vi "Error Handler.vi"(8 "error in":errorcluster, 10 "state":T1=enum."Start", 11 "dispatcher in":refnum<class "Dispatcher Thread.lvclass">) -> (0 "error out":errorcluster, 3 "dispatcher out":refnum<class "Dispatcher Thread.lvclass">)   [LabVIEW 2019, in "DSF Core.lvlib" / "Dispatcher Thread.lvclass"]
uses:
  Dispatcher Thread.lvclass
  Interface/Dispatcher/Command.ctl
  Interface/Dispatcher/Dispatcher Interface.lvclass
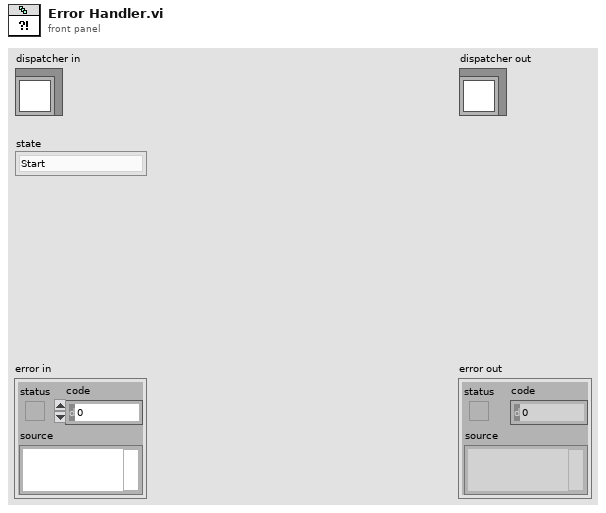
[diagram p1: front panel]
types:
  T1 = typedef "DSF Core.lvlib/Dispatcher Interface.lvclass/Command.ctl" = enum8{"Idle", "Start", "Rx", "Tx", "Set Inline Buffer", "Shutdown", "Error"}
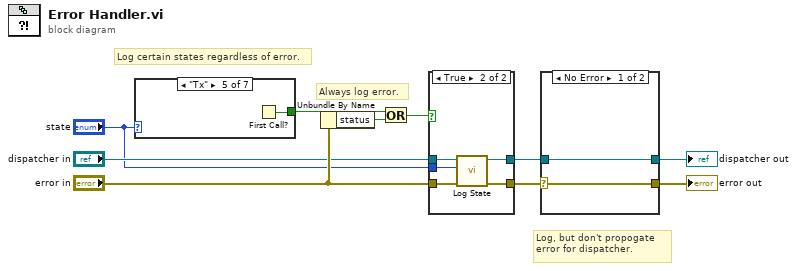
[diagram p0: block diagram]
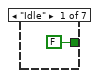
[diagram p2: hidden frame]
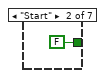
[diagram p3: hidden frame]
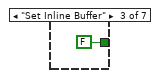
[diagram p4: hidden frame]
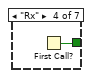
[diagram p5: hidden frame]
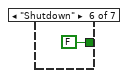
[diagram p6: hidden frame]
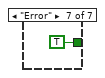
[diagram p7: hidden frame]
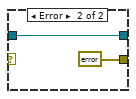
[diagram p9: hidden frame]
diagram:
  # "Log certain states regardless of error."
  # "Always log error."
  # "Log, but don't propogate error for dispatcher."
  n1 = case shown="\"Tx\"" "state" {
    tunnel: [FALSE ("First Call?: T/F") FALSE FALSE ("status") w14 w15 FALSE ("First Call?: T/F") TRUE ("First Call?: T/F")] -> w10
    frame "Idle" {
    }
    frame "Start" {
    }
    frame "Set Inline Buffer" {
    }
    frame "Rx" {
      n2 = First Call?() -> (First Call?: T/F=w14:bool)
    }
    frame "Tx" {
      n3 = First Call?() -> (First Call?: T/F=w15:bool)
    }
    frame "Shutdown" {
    }
    frame "Error" {
    }
  }
  n4 = Unbundle By Name("error in") -> ("status"=w9:bool)
  n5 = Or(x=w10, y=w9) -> (x .or. y?=w8:bool)
  n6 = case shown="True" w8 {
    tunnel: [w19 w21] -> w6
    tunnel: [w18 w20] -> w7
    tunnel: "dispatcher in" -> [w19 w24]
    tunnel: "error in" -> [w18 w23]
    tunnel: "state" -> [_ w22]
    frame False {
    }
    frame True {
      n7 = call "Log State.vi"("error in (no error)"=w23, "state"=w22, "Dispatcher in"=w24) -> ("error out"=w20:errorcluster, "Dispatcher out"=w21:refnum<class "Dispatcher Thread.lvclass">)  [unwired: 7 in]
    }
  }
  n8 = case shown="No Error" w7 {
    selector: w7 -> [w26 _]
    tunnel: w6 -> [w25 w28]
    tunnel: [w26 errorcluster {"status"=FALSE, "code"=0, "source"=""} ("error IO")] -> w1
    tunnel: [w25 w28] -> w2
    frame No Error {
    }
    frame Error {
    }
  }
  "error out" <- w1
  "dispatcher out" <- w2
